vi "MKS670_He3_Main.vi"(7 "stop_external":refnum<vi>, 10 "reference":refnum<vi>, 11 "status_ref":refnum<vi>) -> ()   [LabVIEW 2019]
panel:
  in  "Meas. Interval (ms)":u32=1000
  out "Status":bool
  out "Last Updated":timestamp format="%<%Y-%m-%d %H:%M:%S>T"
  out "Version":dbl
  out "Pressure":waveform(dbl)[](graph)
  in  "Pressure":dbl caption="Torr"
  out "Name":string
  in  "stop":bool
  out "message":string
  in  "GPIB":string="1:8"
  # "MKS Type 670 for He3 Pressure ReadOut"
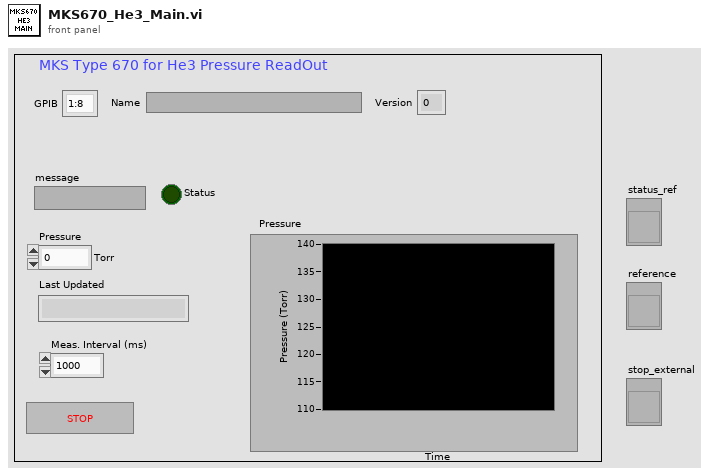
[diagram p1: front panel]
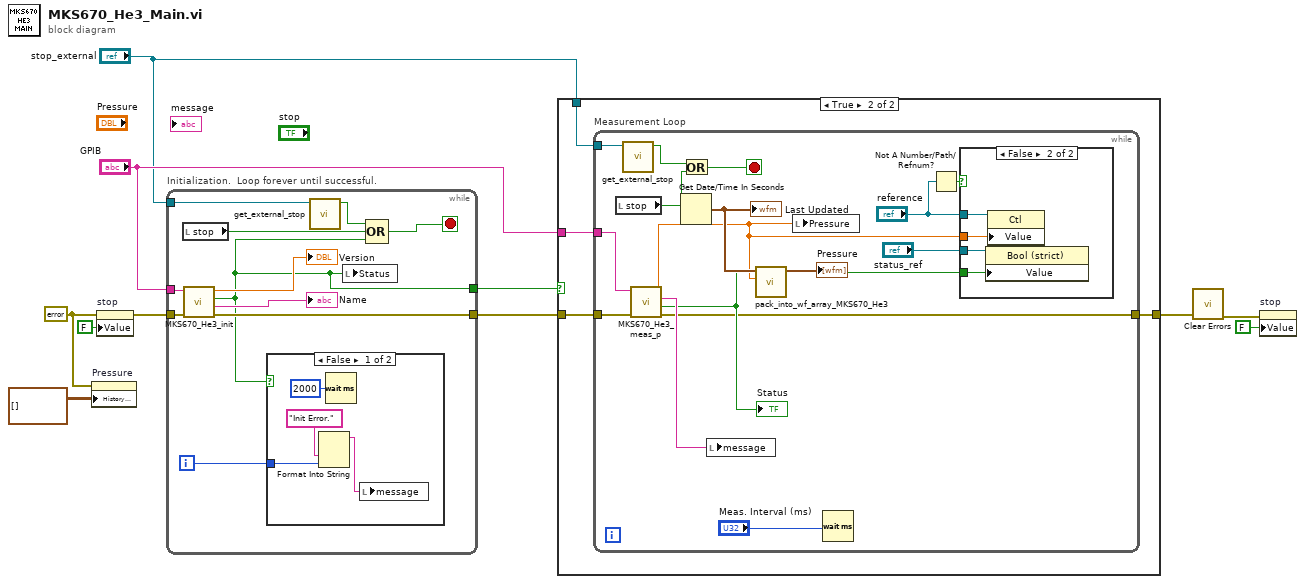
[diagram p0: block diagram]
diagram:
  w7 = errorcluster {"status"=FALSE, "code"=0, "source"=""} ("error in")
  n1 = property on="Pressure" class="WFChart (strict)"(error in=w7, "History Data"=waveform(dbl)[][] []) -> ()  [unwired: 1 in, 2 out]
  n2 = property on="stop" class="Bool (strict)"(error in=w7, "Value"=FALSE ("stop")) -> (error out=w9:errorcluster)  [unwired: 1 in, 1 out]
  n3 = while "Initialization.  Loop forever until successful." {
    tunnel: w9 -> [w21]
    tunnel: "GPIB" -> [w20]
    tunnel: [w19] -> w5
    tunnel: "stop_external" -> [w14]
    tunnel: [w12] -> w4
    i -> [w17]
    stop <- w16 stop-if-true
    n4 = local read "stop"() -> (w15:bool)
    n5 = call "MKS670_He3_init.vi"("error in (no error)"=w21, "GPIB Address"=w20) -> ("error out"=w19:errorcluster, "Device Name"=→"Name":string, "status"=w12:bool, "Device Version"=→"Version":dbl)  [unwired: 6 in]
    n6 = case shown="False" w12 {
      tunnel: w17 -> [w24 _]
      frame False {
        n7 = Format Into String("Init Error.", w24) -> (resulting string=w25:string)  [unwired: 3 in, 1 out]
        n8 = Wait (ms)(milliseconds to wait=u32 2000) -> ()  [unwired: 1 out]
        n9 = local write "message"(w25) -> ()
      }
      frame True {
      }
    }
    n10 = call "get_external_stop.vi"("ref_stop_external"=w14) -> ("stop_output"=w13:bool)  [unwired: 10 in]
    n11 = local write "Status"(w12) -> ()
    n12 = Compound Arithmetic op=OR(w13, w15, w12) -> (w16:bool)
  }
  n13 = case shown="True" w4 {
    tunnel: "GPIB" -> [_ w31]
    tunnel: "stop_external" -> [_ w30]
    tunnel: w5 -> [w27 w29]
    tunnel: [w27 w28] -> w2
    frame False {
    }
    frame True {
      n14 = while "Measurement Loop" {
        tunnel: w31 -> [w47]
        tunnel: w29 -> [w46]
        tunnel: w30 -> [w36]
        tunnel: [w32] -> w28
        stop <- w39 stop-if-true
        n15 = local read "stop"() -> (w37:bool)
        n16 = call "get_external_stop.vi"("ref_stop_external"=w36) -> ("stop_output"=w38:bool)  [unwired: 10 in]
        n17 = call "MKS670_He3_meas_p.vi"("error in"=w46, "GPIB Address"=w47) -> ("error out"=w32:errorcluster, "status"=w34:bool, "msg"=w40:string, "value"=w43:dbl)  [unwired: 6 in]
        "Status" <- w34
        n18 = Get Date/Time In Seconds() -> (seconds since 1Jan1904=w44:timestamp)
        "Last Updated" <- w44
        n19 = Or(x=w38, y=w37) -> (x .or. y?=w39:bool)
        n20 = local write "message"(w40) -> ()
        n21 = call "pack_into_wf_array_MKS670_He3.vi"("pressure"=w43, "time"=w44) -> ("waveform_array"=→"Pressure":waveform(dbl)[])  [unwired: 9 in]
        n22 = local write "Pressure"(w43) -> ()
        n23 = Wait (ms)(milliseconds to wait="Meas. Interval (ms)") -> ()  [unwired: 1 out]
        n24 = Not A Number/Path/Refnum?(number/path/refnum="reference") -> (NaN/Path/Refnum?=w42:bool)
        n25 = case shown="False" w42 {
          tunnel: w43 -> [_ w51]
          tunnel: "reference" -> [_ w50]
          tunnel: "status_ref" -> [_ w49]
          tunnel: w34 -> [_ w48]
          frame True {
          }
          frame False {
            n26 = property class="Bool (strict)"(reference=w49, "Value"=w48) -> ()  [unwired: 1 in, 2 out]
            n27 = property class="Ctl"(reference=w50, "Value"=w51) -> ()  [unwired: 1 in, 2 out]
          }
        }
      }
    }
  }
  n28 = call <vilib>:"Clear Errors.vi"("error in (no error)"=w2) -> ("error out"=w1:errorcluster)  [unwired: 5 in, 1 out]
  n29 = property on="stop" class="Bool (strict)"(error in=w1, "Value"=FALSE ("stop")) -> ()  [unwired: 1 in, 2 out]
